vi "ArmClosedLoopController.vi"(5 "Loop Period":dbl, 6 "Reset I?":bool, 7 "permissable error range":dbl, 8 "I Deadband":dbl=2.0, 9 "Gains":T1, 10 "Cos of Arm Theta":dbl format="%#_13g", 11 "Error":dbl format="%#_13g") -> (1 "PID Variables":cluster{"P":dbl, "I":dbl, "D":dbl, "P+I+D":dbl}, 2 "Device has arrived":bool, 3 "Output":dbl)   [LabVIEW 2014]
uses:
  <vilib>/Analysis/3filter.llb/Filter Passband Type.ctl
  <vilib>/ptbypt/NI_PtbyPt.lvlib
  <vilib>/Analysis/NI_AALBase.lvlib
panel:
  in  "I_Cap":dbl=1.0
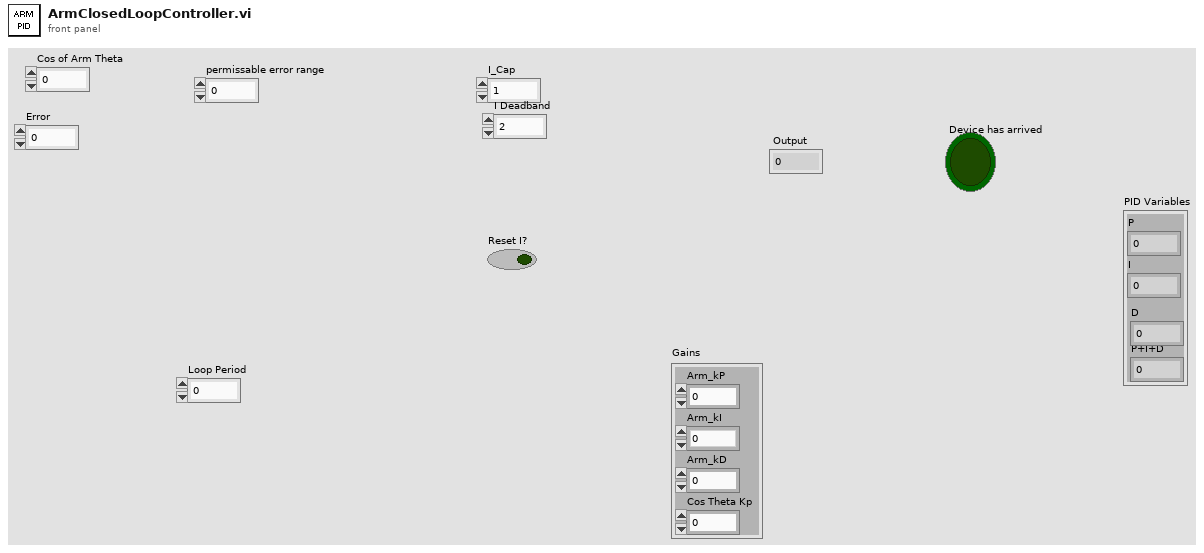
[diagram p1: front panel]
types:
  T1 = cluster{"Arm_kP":dbl, "Arm_kI":dbl, "Arm_kD":dbl, "Cos Theta Kp":dbl}
  T2 = typedef "NI_AALBase.lvlib/Filter Passband Type.ctl" = enum32{"Lowpass", "Highpass", "Bandpass", "Bandstop"}
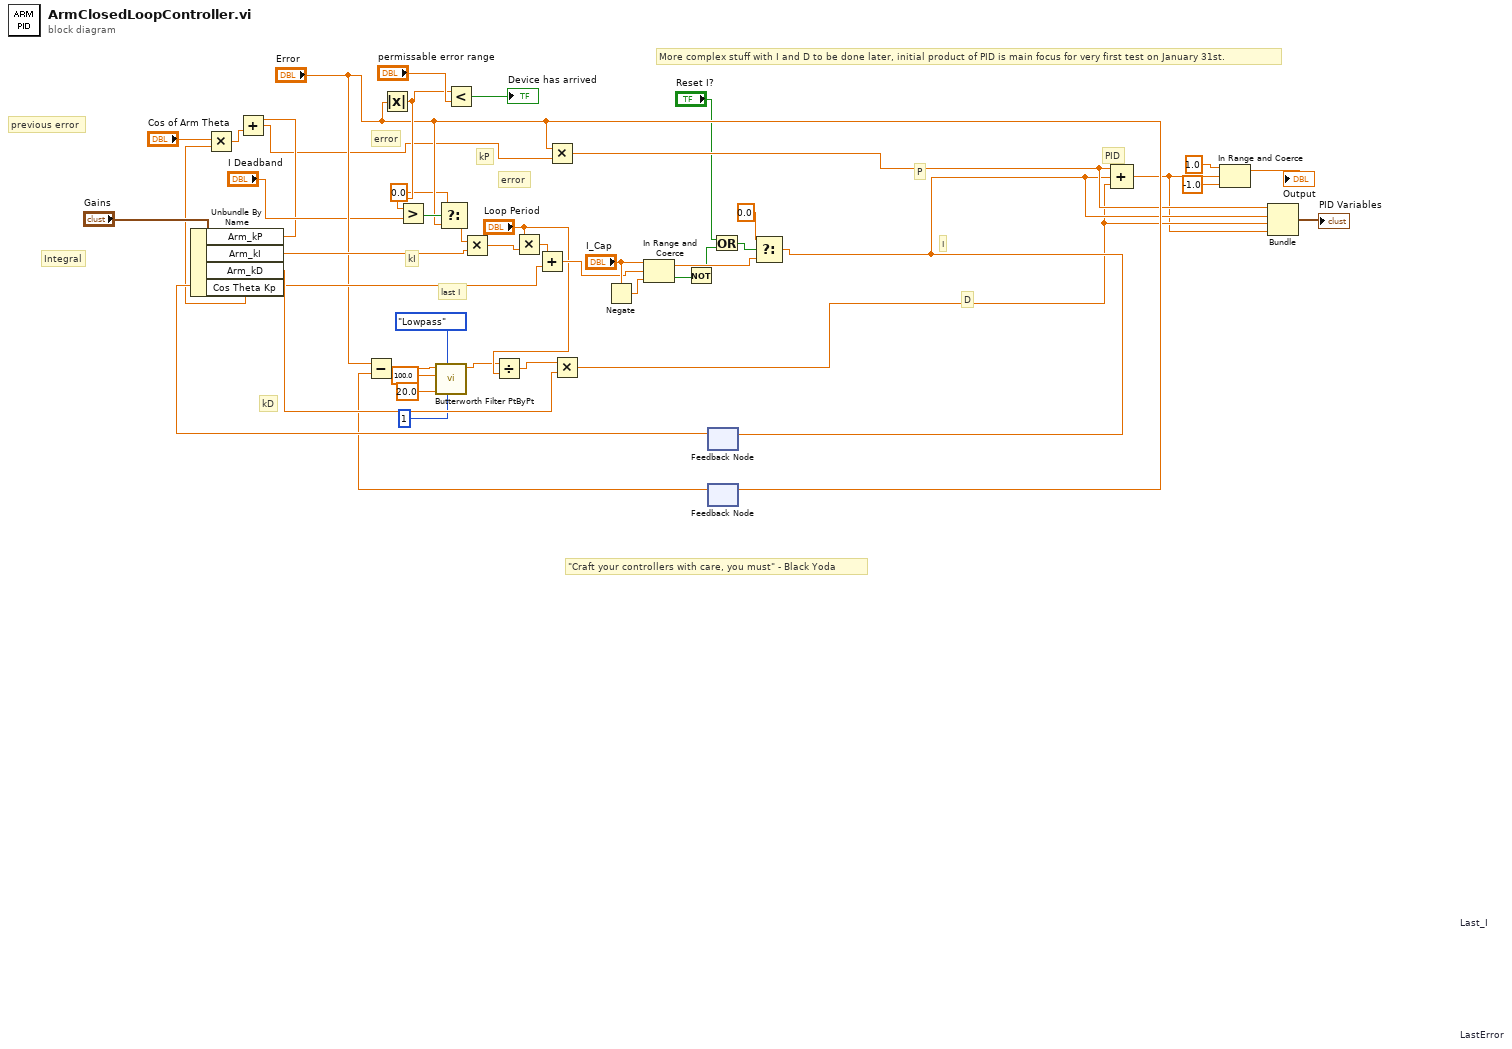
[diagram p0: block diagram]
diagram:
  # "More complex stuff with I and D to be done later, initial product of PID is main focus for very first test on January 31st."
  # "last I"
  # "kI"
  # "error"
  # "kD"
  # "kP"
  # "error"
  # "PID"
  # "D"
  # "I"
  # "P"
  # "Integral"
  # "previous error"
  # "\"Craft your controllers with care, you must\" - Black Yoda"
  n1 = Unbundle By Name("Gains") -> ("Arm_kP"=w2:dbl, "Arm_kI"=w44:dbl, "Arm_kD"=w45:dbl, "Cos Theta Kp"=w5:dbl)
  n2 = Multiply(x="Cos of Arm Theta", y=w5) -> (x*y=w3:dbl)
  n3 = Add(x=w2, y=w3) -> (x+y=w1:dbl)
  n4 = Absolute Value(x="Error") -> (abs(x)=w29:dbl)
  n5 = Greater?(x=w29, y="I Deadband") -> (0:w27:bool)
  n6 = Select(t=0.0, s=w27, f="Error") -> (s? t:f=w28:dbl)
  n7 = Less?(x=w29, y="permissable error range") -> (x < y?=→"Device has arrived":bool)
  n8 = Multiply(x=w28, y=w44) -> (x*y=w30:dbl)
  n9 = Multiply(x="Loop Period", y=w30) -> (x*y=w31:dbl)
  n10 = Multiply(x="Error", y=w1) -> (x*y=w22:dbl)
  n11 = Negate(x="I_Cap") -> (-x=w43:dbl)
  n12 = feedback #1 "Last_I"() -> (w36:dbl)  [unwired: 1 in]
  n13 = Add(x=w31, y=w36) -> (x+y=w39:dbl)
  n14 = In Range and Coerce(upper limit="I_Cap", x=w39, lower limit=w43) -> (coerced(x)=w41:dbl, In Range?=w15:bool)
  n15 = Not(x=w15) -> (.not. x?=w14:bool)
  n16 = feedback #2 "LastError"() -> (w35:dbl)  [unwired: 1 in]
  n17 = Subtract(x="Error", y=w35) -> (x-y=w11:dbl)
  n18 = call <vilib>:"Butterworth Filter PtByPt.vi"("order"=1, "filter type"=Filter_Passband_Type."Lowpass", "low cutoff freq: fl"=20.0, "sampling freq: fs"=100.0, "x"=w11) -> ("Filtered x"=w12:dbl)  [unwired: 4 in, 1 out]
  n19 = Divide(x=w12, y="Loop Period") -> (x/y=w23:dbl)
  n20 = Multiply(x=w23, y=w45) -> (x*y=w20:dbl)
  n21 = feedback-in #2("Error") -> ()
  n22 = Or(x="Reset I?", y=w14) -> (x .or. y?=w17:bool)
  n23 = Select(t=0.0, s=w17, f=w41) -> (s? t:f=w21:dbl)
  n24 = feedback-in #1(w21) -> ()
  n25 = Compound Arithmetic op=ADD(w22, w21, w20) -> (w19:dbl)
  n26 = In Range and Coerce(upper limit=1.0, x=w19, lower limit=-1.0) -> (coerced(x)=→"Output":dbl)  [unwired: 1 out]
  n27 = Bundle(w22, "I_Cap"=w21, w20, w19) -> (→"PID Variables":cluster{dbl, "I_Cap":dbl, dbl, dbl})  [unwired: 1 in]
